vi "FestoCPX.Station.ProdLift.CheckSlot.vi"(8 "error in":errorcluster, 11 "Slot":T1) -> (0 "error out":errorcluster, 1 "Work":bool, 2 "Home":bool)   [LabVIEW 2016]
uses:
  Station/Station.ProductSlot.ctl
  FestoCPX.DI.Signal.ctl
  FestoCPX.DO.Signal.ctl
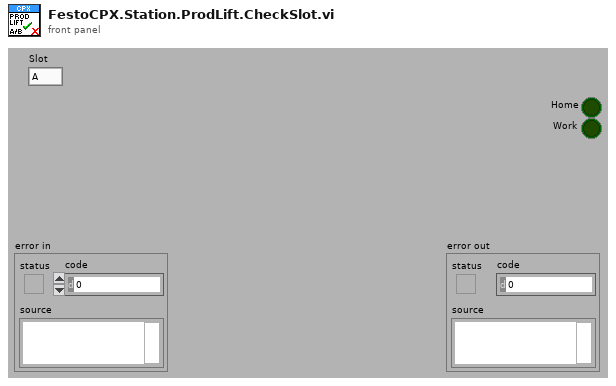
[diagram p1: front panel]
types:
  T1 = typedef "Station.ProductSlot.ctl" = enum8{"A", "B"}
  T2 = typedef "FestoCPX.DO.Signal.ctl" = enum16{"Safety Reset", "Air Main Valve", "Door Lock", "Button LED Start", "Button LED Stop", "Button LED Control", "Traffic LED Red", "Traffic LED Orange", "Traffic LED Green", "Horn", "Laser Interlock", "Laser Trigger", "Laser Fume Extractor", "Product Suction Gripper Slot 1 A", "Product Suction Gripper Slot 1 B", "Product Suction Gripper Slot 2 A", "Product Suction Gripper Slot 2 B", "Product Suction Gripper Slot 3 A", "Product Suction Gripper Slot 3 B", "Product Suction Gripper Slot 4 A", "Product Suction Gripper Slot 4 B", "Product Suction Gripper Final A", "Product Suction Gripper Final B", "Lamp", "Q1 Product Move Work", "Q1 Product Move Home", "Q2 Table Turn Work", "Q2 Table Turn Home", "Q3 Product Lift A", "Q3 Product Lift B", "Q4 Product Arm OK", "Q4 Product Arm NOK", "Q5 Product Arm Work", "Q6 Product BlowOut A", "Q6 Product BlowOut B"}
  T3 = typedef "FestoCPX.DI.Signal.ctl" = enum16{"S.C. Emergency Stop", "S.C. Side Door Close", "S.C. Front Door Close", "S.C. Front Door Secured", "Button Start", "Button Stop", "Button Control", "Product Move Home", "Product Move Work", "Table Position", "Table Lock", "Product Lift A Home", "Product Lift B Home", "Product Arm OK", "Product Arm NOK", "Product Arm Work", "Revolver ID 1", "Revolver ID 2", "Revolver ID 3", "Revolver ID 4", "Revolver ID 5", "Air Pressure Inside", "Air Pressure Inlet", "Product Slot 1 A Present", "Product Slot 1 B Present", "Product Slot 2 A Present", "Product Slot 2 B Present", "Product Slot 3 A Present", "Product Slot 3 B Present", "Product Slot 4 A Present", "Product Slot 4 B Present", "Product Final A Present", "Product Final B Present", "Product Output A Present", "Product Output B Present", "Product Container OK Present", "Product Container NOK Present", "Fork ID 1", "Fork ID 2"}
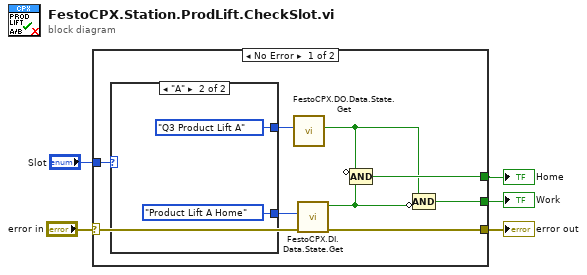
[diagram p0: block diagram]
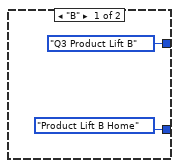
[diagram p2: hidden frame]
diagram:
  n1 = case shown="No Error" "error in" {
    selector: "error in" -> [w14 w19]
    tunnel: [w13 w19] -> w5
    tunnel: [w9 _] -> w2
    tunnel: [w8 _] -> w1
    tunnel: "Slot" -> [w10 _]
    frame No Error {
      n2 = case shown="\"A\"" w10 {
        tunnel: [FestoCPX.DI.Signal."Product Lift B Home" ("DI") FestoCPX.DI.Signal."Product Lift A Home" ("DI")] -> w12
        tunnel: [FestoCPX.DO.Signal."Q3 Product Lift B" ("CPX.DO") FestoCPX.DO.Signal."Q3 Product Lift A" ("CPX.DO")] -> w11
        frame "B" {
        }
        frame "A" {
        }
      }
      n3 = call "FestoCPX.DO.Data.State.Get.vi"("CPX.DO"=w11) -> ("State"=w7:bool)  [unwired: 9 in, 1 out]
      n4 = call "FestoCPX.DI.Data.State.Get.vi"("error in (no error)"=w14, "CPX.DI"=w12) -> ("error out"=w13:errorcluster, "State"=w6:bool)  [unwired: 5 in, 3 out]
      n5 = Compound Arithmetic op=AND(invert w7, w6) -> (w9:bool)
      n6 = Compound Arithmetic op=AND(w7, invert w6) -> (w8:bool)
    }
    frame Error {
    }
  }
  "error out" <- w5
  "Work" <- w1
  "Home" <- w2
